vi "Sensors-Light uno.vi"() -> ()   [LabVIEW 2011]
uses:
  <vilib>/LabVIEW Interface for Arduino/Type Defs/Board Type.ctl
  <vilib>/LabVIEW Interface for Arduino/Type Defs/LCD Pin Config 4 bit.ctl
  <vilib>/LabVIEW Interface for Arduino/Type Defs/Direction.ctl
  <vilib>/LabVIEW Interface for Arduino/Type Defs/Pin Mode.ctl
  <vilib>/LabVIEW Interface for Arduino/LabVIEW Interface for Arduino.lvlib
panel:
  in  "stop":bool
  in  "stop 10":bool
  out "NEW VALUE":string="Hello World"
  in  "stop 8":bool
  out "Alarm Led":bool
  in  "stop 7":bool
  out "RGB":u32(colorbox)
  in  "stop 6":bool
  out "Entree Light":bool
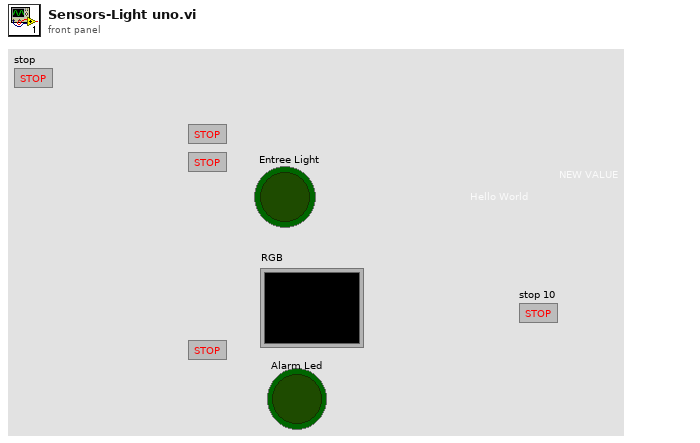
[diagram p1: front panel]
types:
  T1 = typedef "LabVIEW Interface for Arduino.lvlib/Board Type.ctl" = enum16{"Uno", "Dimuelanove w/Atmega 328", "Mega 2560"}
  T2 = typedef "LabVIEW Interface for Arduino.lvlib/Arduino Resource.ctl" = cluster{"VISA resource":refnum<visa-resource-name>, "Board Type":T1, "Connection Type":enum8{"USB / Serial"}, "Bytes Per Packet (15)":u8}
  T3 = typedef "LabVIEW Interface for Arduino.lvlib/LCD Pin Config 4 bit.ctl" = cluster{"RS":u8, "RW":u8, "Enable":u8, "D4":u8, "D5":u8, "D6":u8, "D7":u8, "LCD":u8}
  T4 = typedef "LabVIEW Interface for Arduino.lvlib/Direction.ctl" = enum8{"Left ", "Right"}
  T5 = enum8{"String", "Binary", "Decimal", "Octal", "Hexadecimal"}
  T6 = typedef "LabVIEW Interface for Arduino.lvlib/Pin Mode.ctl" = enum8{"Input", "Output"}
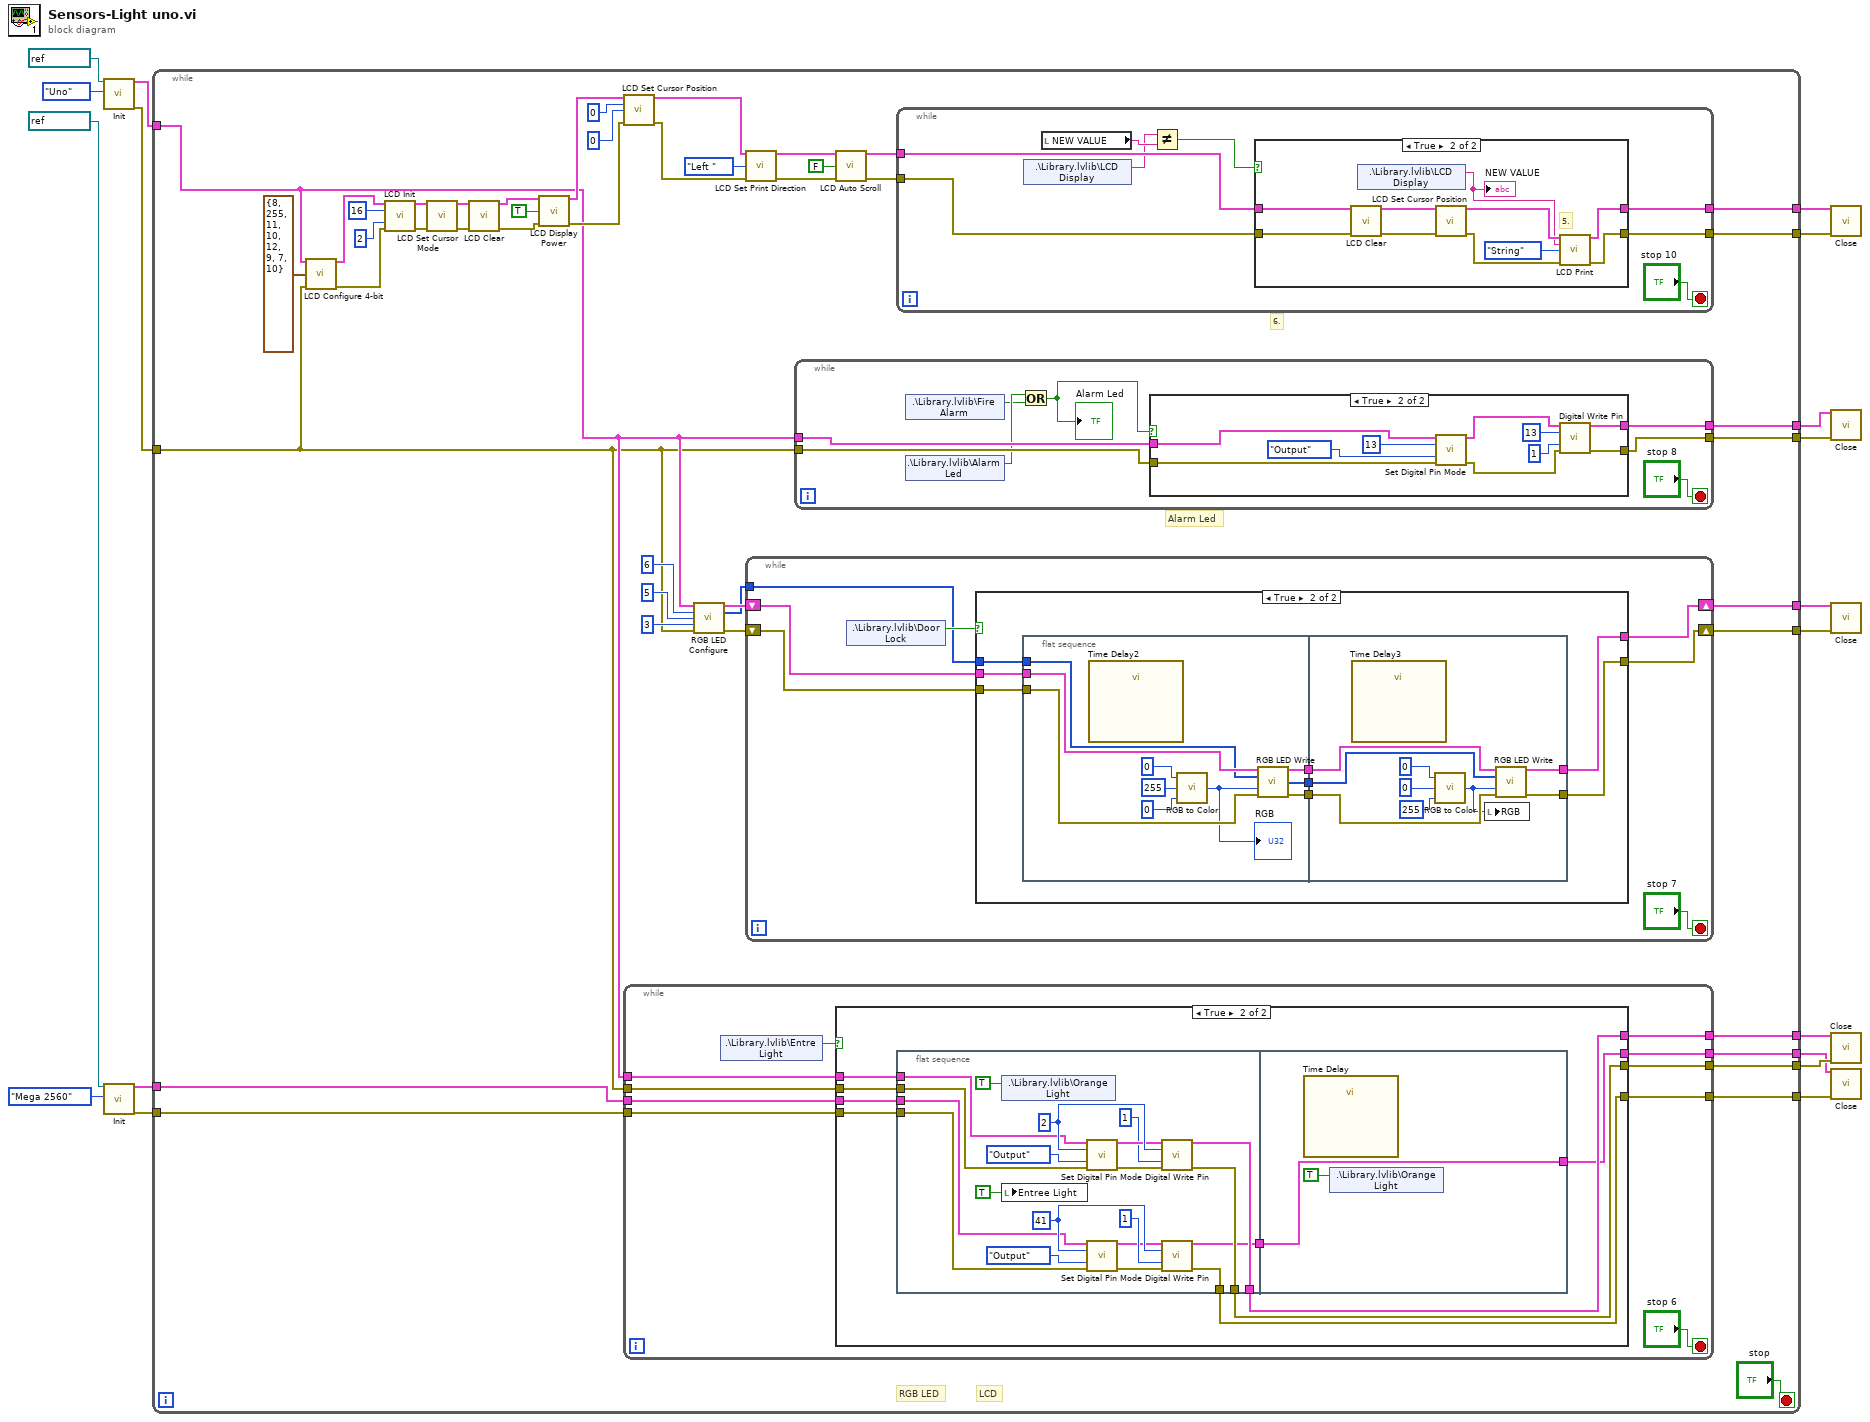
[diagram p0: block diagram]
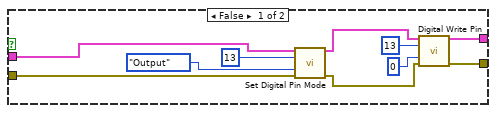
[diagram p3: hidden frame]
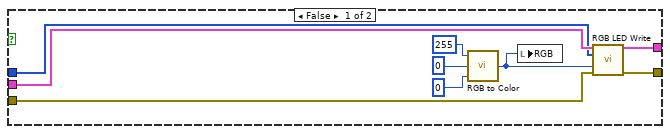
[diagram p4: hidden frame]
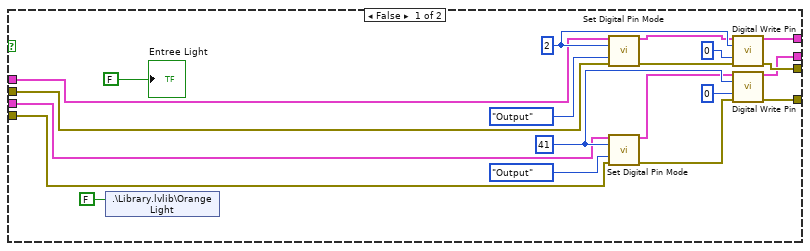
[diagram p5: hidden frame]
diagram:
  n1 = call <vilib>:"Init.vi"("VISA resource"=refnum<visa-resource-name> "COM3", "Board Type (Uno)"=Board_Type."Uno") -> ("Arduino Resource"=w16:T2, "error out"=w15:errorcluster)  [unwired: 16 in]
  n2 = call <vilib>:"Init.vi"("VISA resource"=refnum<visa-resource-name> "COM4", "Board Type (Uno)"=Board_Type."Mega 2560") -> ("Arduino Resource"=w6:T2, "error out"=w5:errorcluster)  [unwired: 16 in]
  n3 = while {
    tunnel: w16 -> [w21]
    tunnel: w15 -> [w20]
    tunnel: [w57] -> w14
    tunnel: [w56] -> w13
    tunnel: [w55] -> w12
    tunnel: [w54] -> w11
    tunnel: [w53] -> w10
    tunnel: [w52] -> w9
    tunnel: w6 -> [w51]
    tunnel: w5 -> [w50]
    tunnel: [w49] -> w4
    tunnel: [w48] -> w3
    tunnel: [w23] -> w2
    tunnel: [w22] -> w1
    stop <- "stop" stop-if-true
    # "6."
    # "LCD"
    # "Alarm Led"
    # "RGB LED"
    n4 = call <vilib>:"LCD Configure 4-bit.vi"("Arduino Resource"=w21, "LCD Pin Config 4 Bit"=T3 {"RS"=8, "RW"=255, "Enable"=11, "D4"=10, "D5"=12, "D6"=9, "D7"=7, "LCD"=10}, "error in"=w20) -> ("Arduino Resource"=w30:T2, "error out"=w29:errorcluster)  [unwired: 11 in]
    n5 = call <vilib>:"LCD Init.vi"("Arduino Resource"=w30, "Columns"=u8 16, "Rows"=u8 2, "error in"=w29) -> ("Arduino Resource"=w40:T2, "error out"=w39:errorcluster)  [unwired: 10 in]
    n6 = call <vilib>:"LCD Set Cursor Mode.vi"("Arduino Resource"=w40, "error out"=w39) -> ("Arduino Resource"=w38:T2, "error out"=w37:errorcluster)  [unwired: 12 in]
    n7 = call <vilib>:"LCD Clear.vi"("Arduino Resource"=w38, "error in"=w37) -> ("Arduino Resource"=w41:T2, "error out"=w42:errorcluster)  [unwired: 12 in]
    n8 = call <vilib>:"LCD Display Power.vi"("Arduino Resource"=w41, "Display On? (T) 2"=TRUE, "error in"=w42) -> ("Arduino Resource"=w44:T2, "error out"=w45:errorcluster)  [unwired: 11 in]
    n9 = call <vilib>:"LCD Set Cursor Position.vi"("Arduino Resource"=w44, "Column"=u8 0, "Row"=u8 0, "error out"=w45) -> ("Arduino Resource"=w35:T2, "error out"=w34:errorcluster)  [unwired: 10 in]
    n10 = while {
      tunnel: w21 -> [w162]
      tunnel: w20 -> [w161]
      tunnel: [w160] -> w57
      tunnel: [w159] -> w56
      tunnel: w51 -> [w158]
      tunnel: w50 -> [w157]
      tunnel: [w156] -> w49
      tunnel: [w155] -> w48
      stop <- "stop 6" stop-if-true
      n11 = shared-variable ".\\Library.lvlib\\Entre Light"() -> (w163:bool)  [unwired: 1 in, 1 out]
      n12 = case shown="True" w163 {
        tunnel: w162 -> [w179 w193]
        tunnel: w161 -> [w178 w192]
        tunnel: [w177 w191] -> w160
        tunnel: [w176 w190] -> w159
        tunnel: w158 -> [w168 w189]
        tunnel: w157 -> [w167 w188]
        tunnel: [w166 w187] -> w156
        tunnel: [w165 w185] -> w155
        frame False {
          w172 = u8 41 ("Digital I/O Pin")
          w184 = u8 2 ("Digital I/O Pin")
          n13 = shared-variable ".\\Library.lvlib\\Orange Light"(FALSE ("Orange Light")) -> ()  [unwired: 1 in, 1 out]
          n14 = call <vilib>:"Set Digital Pin Mode.vi"("Arduino Resource"=w179, "Digital I/O Pin"=w184, "Pin Mode (Input)"=Pin_Mode."Output", "error in"=w178) -> ("Arduino Resource"=w182:T2, "error out"=w183:errorcluster)  [unwired: 10 in]
          n15 = call <vilib>:"Set Digital Pin Mode.vi"("Arduino Resource"=w168, "Digital I/O Pin"=w172, "Pin Mode (Input)"=Pin_Mode."Output", "error in"=w167) -> ("Arduino Resource"=w169:T2, "error out"=w170:errorcluster)  [unwired: 10 in]
          n16 = call <vilib>:"Digital Write Pin.vi"("Arduino Resource"=w182, "Digital I/O Pin (0)"=w184, "Value (0)"=u8 0, "error in"=w183) -> ("Arduino Resource"=w177:T2, "error out"=w176:errorcluster)  [unwired: 10 in]
          n17 = call <vilib>:"Digital Write Pin.vi"("Arduino Resource"=w169, "Digital I/O Pin (0)"=w172, "Value (0)"=u8 0, "error in"=w170) -> ("Arduino Resource"=w166:T2, "error out"=w165:errorcluster)  [unwired: 10 in]
          "Entree Light" <- FALSE ("Entree Light")
        }
        frame True {
          n18 = flat-sequence {
            tunnel: w193 -> [w209]
            tunnel: w192 -> [w208]
            tunnel: [w207] -> w191
            tunnel: [w206] -> w190
            tunnel: w189 -> [w197]
            tunnel: w188 -> [w196]
            tunnel: [w195] -> w186
            tunnel: [w194] -> w185
            tunnel: [w214] -> w187
            tunnel: w186 -> [w214]
            frame #0 {
              w201 = u8 41 ("Digital I/O Pin")
              w213 = u8 2 ("Digital I/O Pin")
              n19 = shared-variable ".\\Library.lvlib\\Orange Light"(TRUE ("Orange Light")) -> ()  [unwired: 1 in, 1 out]
              n20 = local write "Entree Light"(TRUE ("Entree Light")) -> ()
              n21 = call <vilib>:"Set Digital Pin Mode.vi"("Arduino Resource"=w209, "Digital I/O Pin"=w213, "Pin Mode (Input)"=Pin_Mode."Output", "error in"=w208) -> ("Arduino Resource"=w211:T2, "error out"=w212:errorcluster)  [unwired: 10 in]
              n22 = call <vilib>:"Set Digital Pin Mode.vi"("Arduino Resource"=w197, "Digital I/O Pin"=w201, "Pin Mode (Input)"=Pin_Mode."Output", "error in"=w196) -> ("Arduino Resource"=w198:T2, "error out"=w199:errorcluster)  [unwired: 10 in]
              n23 = call <vilib>:"Digital Write Pin.vi"("Arduino Resource"=w211, "Digital I/O Pin (0)"=w213, "Value (0)"=u8 1, "error in"=w212) -> ("Arduino Resource"=w207:T2, "error out"=w206:errorcluster)  [unwired: 10 in]
              n24 = call <vilib>:"Digital Write Pin.vi"("Arduino Resource"=w198, "Digital I/O Pin (0)"=w201, "Value (0)"=u8 1, "error in"=w199) -> ("Arduino Resource"=w195:T2, "error out"=w194:errorcluster)  [unwired: 10 in]
            }
            frame #1 {
              n25 = call "Time Delay"() -> ()  [unwired: 11 in, 1 out]
              n26 = shared-variable ".\\Library.lvlib\\Orange Light"(TRUE ("Orange Light")) -> ()  [unwired: 1 in, 1 out]
            }
          }
        }
      }
    }
    n27 = call <vilib>:"RGB LED Configure.vi"("Arduino Resource"=w21, "Red Pin"=u8 6, "Green Pin"=u8 5, "Blue Pin"=u8 3, "error in"=w20) -> ("Arduino Resource"=w63:T2, "RGB LED Pins"=w58:u8[], "error out"=w62:errorcluster)  [unwired: 8 in]
    n28 = call <vilib>:"LCD Set Print Direction.vi"("Arduino Resource"=w35, "Print Direction"=Direction."Left " ("Direction"), "error in"=w34) -> ("Arduino Resource"=w32:T2, "error"=w31:errorcluster)  [unwired: 11 in]
    n29 = while {
      shift-right: [w113] -> w55
      shift-left: w63 -> [w116]
      shift-right: [w112] -> w54
      shift-left: w62 -> [w114]
      tunnel: w58 -> [w115]
      stop <- "stop 7" stop-if-true
      n30 = shared-variable ".\\Library.lvlib\\Door Lock"() -> (w117:bool)  [unwired: 1 in, 1 out]
      n31 = case shown="True" w117 {
        tunnel: w116 -> [w124 w135]
        tunnel: w115 -> [w123 w134]
        tunnel: w114 -> [w122 w133]
        tunnel: [w121 w129] -> w113
        tunnel: [w120 w128] -> w112
        frame False {
          n32 = call <vilib>:"RGB to Color.vi"("B"=u8 0, "G"=u8 0, "R"=u8 255) -> ("Color"=w119:u32)
          n33 = local write "RGB"(w119) -> ()
          n34 = call <vilib>:"RGB LED Write.vi"("Arduino Resource"=w124, "RGB LED Pins"=w123, "Color"=w119, "error in"=w122) -> ("Arduino Resource"=w121:T2, "error out"=w120:errorcluster)  [unwired: 9 in, 1 out]
        }
        frame True {
          n35 = flat-sequence {
            tunnel: w135 -> [w145]
            tunnel: w134 -> [w144]
            tunnel: w133 -> [w143]
            tunnel: [w139] -> w132
            tunnel: [w138] -> w131
            tunnel: [w137] -> w130
            tunnel: w132 -> [w154]
            tunnel: w131 -> [w153]
            tunnel: w130 -> [w152]
            tunnel: [w148] -> w129
            tunnel: [w147] -> w128
            frame #0 {
              n36 = call "Time Delay2"() -> ()  [unwired: 11 in, 1 out]
              n37 = call <vilib>:"RGB to Color.vi"("B"=u8 0, "G"=u8 255, "R"=u8 0) -> ("Color"=w136:u32)
              "RGB" <- w136
              n38 = call <vilib>:"RGB LED Write.vi"("Arduino Resource"=w145, "RGB LED Pins"=w144, "Color"=w136, "error in"=w143) -> ("Arduino Resource"=w139:T2, "RGB LED Pins Out"=w137:u8[], "error out"=w138:errorcluster)  [unwired: 9 in]
            }
            frame #1 {
              n39 = call "Time Delay3"() -> ()  [unwired: 11 in, 1 out]
              n40 = call <vilib>:"RGB to Color.vi"("B"=u8 255 ("G"), "G"=u8 0 ("B"), "R"=u8 0) -> ("Color"=w146:u32)
              n41 = local write "RGB"(w146) -> ()
              n42 = call <vilib>:"RGB LED Write.vi"("Arduino Resource"=w154, "RGB LED Pins"=w152, "Color"=w146, "error in"=w153) -> ("Arduino Resource"=w148:T2, "error out"=w147:errorcluster)  [unwired: 9 in, 1 out]
            }
          }
        }
      }
    }
    n43 = while {
      tunnel: w21 -> [w90]
      tunnel: [w89] -> w53
      tunnel: [w88] -> w52
      tunnel: w20 -> [w87]
      stop <- "stop 8" stop-if-true
      n44 = shared-variable ".\\Library.lvlib\\Fire Alarm"() -> (w85:bool)  [unwired: 1 in, 1 out]
      n45 = shared-variable ".\\Library.lvlib\\Alarm Led"() -> (w86:bool)  [unwired: 1 in, 1 out]
      n46 = Or(x=w86, y=w85) -> (x .or. y?=w84:bool)
      "Alarm Led" <- w84
      n47 = case shown="True" w84 {
        tunnel: w90 -> [w93 w104]
        tunnel: [w95 w111] -> w89
        tunnel: [w94 w110] -> w88
        tunnel: w87 -> [w92 w105]
        frame False {
          n48 = call <vilib>:"Set Digital Pin Mode.vi"("Arduino Resource"=w93, "Digital I/O Pin"=u8 13, "Pin Mode (Input)"=Pin_Mode."Output", "error in"=w92) -> ("Arduino Resource"=w99:T2, "error out"=w98:errorcluster)  [unwired: 10 in]
          n49 = call <vilib>:"Digital Write Pin.vi"("Arduino Resource"=w99, "Digital I/O Pin (0)"=u8 13, "Value (0)"=u8 0, "error in"=w98) -> ("Arduino Resource"=w95:T2, "error out"=w94:errorcluster)  [unwired: 10 in]
        }
        frame True {
          n50 = call <vilib>:"Set Digital Pin Mode.vi"("Arduino Resource"=w104, "Digital I/O Pin"=u8 13, "Pin Mode (Input)"=Pin_Mode."Output", "error in"=w105) -> ("Arduino Resource"=w107:T2, "error out"=w106:errorcluster)  [unwired: 10 in]
          n51 = call <vilib>:"Digital Write Pin.vi"("Arduino Resource"=w107, "Digital I/O Pin (0)"=u8 13, "Value (0)"=u8 1, "error in"=w106) -> ("Arduino Resource"=w111:T2, "error out"=w110:errorcluster)  [unwired: 10 in]
        }
      }
    }
    n52 = call <vilib>:"LCD Auto Scroll.vi"("Arduino Resource"=w32, "Auto Scroll?"=FALSE ("Auto Scroll? 2"), "error in"=w31) -> ("Arduino Resource"=w25:T2, "error out"=w24:errorcluster)  [unwired: 11 in]
    n53 = while {
      tunnel: [w71] -> w23
      tunnel: [w70] -> w22
      tunnel: w25 -> [w66]
      tunnel: w24 -> [w65]
      stop <- "stop 10" stop-if-true
      n54 = shared-variable ".\\Library.lvlib\\LCD Display"() -> (w64:string)  [unwired: 1 in, 1 out]
      n55 = local read "NEW VALUE"() -> (w68:string)
      n56 = Not Equal?(x=w64, y=w68) -> (x != y?=w67:bool)
      n57 = case shown="True" w67 {
        tunnel: [w73 w78] -> w71
        tunnel: [w72 w77] -> w70
        tunnel: w66 -> [w73 w76]
        tunnel: w65 -> [w72 w75]
        frame False {
        }
        frame True {
          # "5."
          n58 = call <vilib>:"LCD Clear.vi"("Arduino Resource"=w76, "error in"=w75) -> ("Arduino Resource"=w83:T2, "error out"=w82:errorcluster)  [unwired: 12 in]
          n59 = shared-variable ".\\Library.lvlib\\LCD Display"() -> (w74:string)  [unwired: 1 in, 1 out]
          "NEW VALUE" <- w74
          n60 = call <vilib>:"LCD Set Cursor Position.vi"("Arduino Resource"=w83, "error out"=w82) -> ("Arduino Resource"=w81:T2, "error out"=w80:errorcluster)  [unwired: 12 in]
          n61 = call <vilib>:"LCD Print.vi"("Arduino Resource"=w81, "Data"=w74, "Base (String)"=T5."String", "error out"=w80) -> ("Arduino Resource"=w78:T2, "error out"=w77:errorcluster)  [unwired: 10 in]
        }
      }
    }
  }
  n62 = call <vilib>:"Close.vi"("Arduino Resource"=w2, "error in"=w1) -> ()  [unwired: 13 in, 1 out]
  n63 = call <vilib>:"Close.vi"("Arduino Resource"=w10, "error in"=w9) -> ()  [unwired: 13 in, 1 out]
  n64 = call <vilib>:"Close.vi"("Arduino Resource"=w12, "error in"=w11) -> ()  [unwired: 13 in, 1 out]
  n65 = call <vilib>:"Close.vi"("Arduino Resource"=w14, "error in"=w13) -> ()  [unwired: 13 in, 1 out]
  n66 = call <vilib>:"Close.vi"("Arduino Resource"=w4, "error in"=w3) -> ()  [unwired: 13 in, 1 out]
